vi "GetFileTrajectoFTP.vi"(4 "error in (no error)":errorcluster caption="entrée d'erreur (pas d'erreur)", 6 "NewTrajectoFile":path, 7 "NomProjet":string) -> (0 "error out":errorcluster caption="sortie d'erreur", 3 "NomProjetOut":string)   [LabVIEW 2017]
uses:
  <vilib>/FTP/NI_FTP.lvlib
panel:
  out "remotePath":string
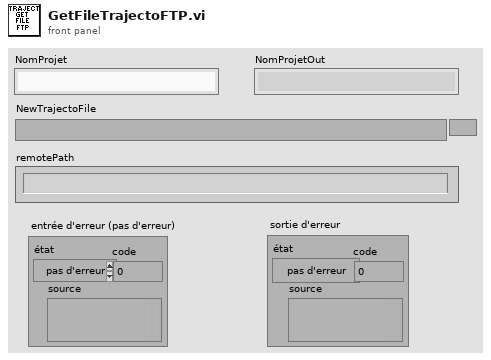
[diagram p1: front panel]
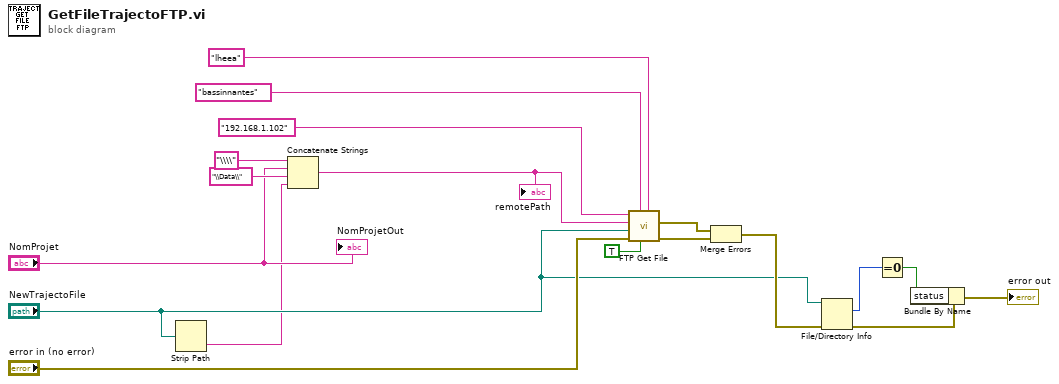
[diagram p0: block diagram]
diagram:
  n1 = Strip Path(path="NewTrajectoFile") -> (name=w1:string)  [unwired: 1 out]
  n2 = Concatenate Strings("\\\\" ("chaîne"), "NomProjet", "\\Data\\" ("chaîne"), w1) -> (w10:string)
  "remotePath" <- w10
  n3 = call <vilib>:"FTP Get File.vi"("password"="lheea", "binary (F)"=TRUE, "user"="bassinnantes", "error in (no error)"="error in (no error)", "local path"="NewTrajectoFile", "remote path"=w10, "host"="192.168.1.102") -> ("error out"=w13:errorcluster, "file error"=w14:errorcluster)  [unwired: 3 in]
  n4 = Merge Errors(w14, w13) -> (w9:errorcluster)
  n5 = File/Directory Info(path="NewTrajectoFile", error in=w9) -> (size=w8:i64, error out=w5:errorcluster)  [unwired: 5 out]
  n6 = Equal To 0?(x=w8) -> (x = 0?=w7:bool)
  n7 = Bundle By Name(cluster=w5, "status"=w7) -> (→"error out":errorcluster)
  "NomProjetOut" <- "NomProjet"
